vi "Self-Test.vi"(0 "VISA resource name":refnum<visa-resource-name>, 11 "error in (no error)":errorcluster {"code" format="%.0x"}) -> (4 "VISA resource name out":refnum<visa-resource-name>, 8 "Self-Test Result Code":i32, 10 "Self-Test Result Message":string, 15 "error out":errorcluster {"code" format="%.0x"})   [LabVIEW 2010, in "Agilent N6700 Series.lvlib"]
doc: "This VI runs the instrument's self test routine and returns the test results."
uses:
  Agilent N6700 Series.lvlib
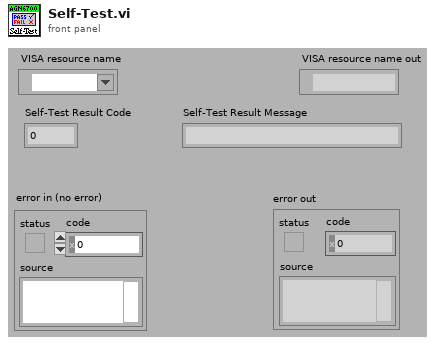
[diagram p1: front panel]
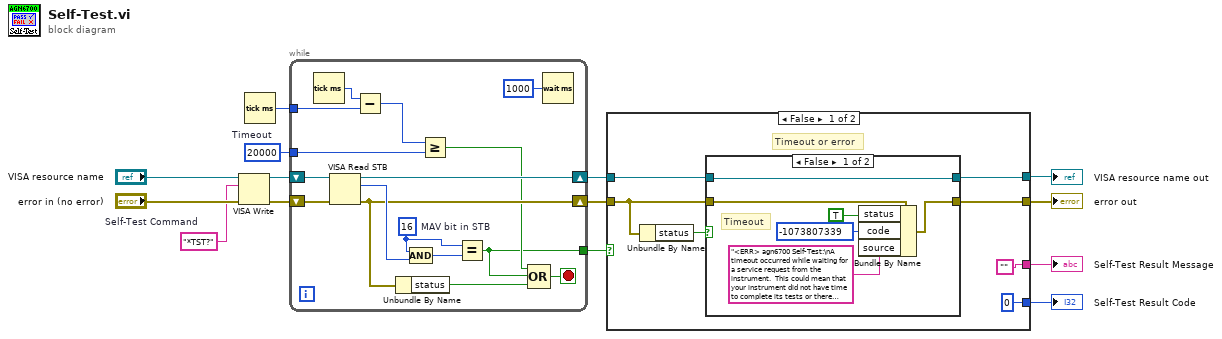
[diagram p0: block diagram]
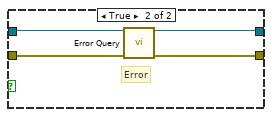
[diagram p2: hidden frame]
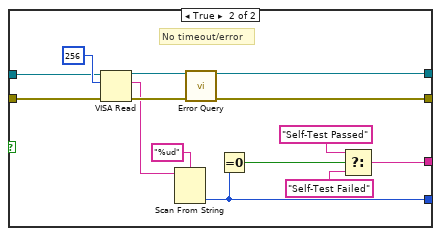
[diagram p3: hidden frame]
diagram:
  w2 = u32 20000  # Timeout
  w11 = "*TST?"  # Self-Test Command
  n1 = VISA Write(VISA resource name="VISA resource name", write buffer=w11, error in (no error)="error in (no error)") -> (VISA resource name out=w10:refnum<visa-resource-name>, error out=w9:errorcluster)  [unwired: 1 out]
  n2 = Tick Count (ms)() -> (millisecond timer value=w3:u32)
  n3 = while {
    shift-right: [w23] -> w7
    shift-left: w9 -> [w27]
    shift-right: [w25] -> w8
    shift-left: w10 -> [w26]
    tunnel: w3 -> [w19]
    tunnel: w2 -> [w17]
    tunnel: [w15] -> w1
    stop <- w21 stop-if-true
    w30 = u16 16  # MAV bit in STB
    n4 = Tick Count (ms)() -> (millisecond timer value=w20:u32)
    n5 = VISA Read STB(8:w27, 11:w26) -> (0:w23:errorcluster, 2:w28:u16, 3:w25:refnum<visa-resource-name>)
    n6 = Subtract(x=w20, y=w19) -> (x-y=w18:u32)
    n7 = Unbundle By Name(w23) -> ("status"=w22:bool)
    n8 = Compound Arithmetic op=AND(w30, w28) -> (w29:u16)
    n9 = Greater Or Equal?(x=w18, y=w17) -> (x >= y?=w16:bool)
    n10 = Equal?(x=w30, y=w29) -> (x = y?=w15:bool)
    n11 = Compound Arithmetic op=OR(w16, w15, w22) -> (w21:bool)
    n12 = Wait (ms)(milliseconds to wait=u32 1000) -> ()  [unwired: 1 out]
  }
  n13 = case shown="False" w1 {
    tunnel: ["" w48] -> w14
    tunnel: w8 -> [w36 w60]
    tunnel: w7 -> [w34 w59]
    tunnel: [0 w52] -> w6
    tunnel: [w35 w55] -> w5
    tunnel: [w33 w54] -> w4
    frame False {
      # "Timeout or error"
      n14 = Unbundle By Name(w34) -> ("status"=w37:bool)
      n15 = case shown="False" w37 {
        tunnel: w36 -> [w38 w47]
        tunnel: [w38 w44] -> w35
        tunnel: [w39 w45] -> w33
        tunnel: w34 -> [w40 w46]
        frame False {
          # "Timeout"
          n16 = Bundle By Name(cluster=w40, "status"=TRUE, "code"=-1073807339, "source"="<ERR> agn6700 Self-Test:\nA timeout occurred while waiting for a service request from the instrument.  This could mean that your instrument did not have time to complete its tests or there could be a problem communicating with the instrument.") -> (w39:errorcluster)
        }
        frame True {
          # "Error"
          n17 = call "Error Query.vi"("VISA resource name"=w47, "error in (no error)"=w46) -> ("VISA resource name out"=w44:refnum<visa-resource-name>, "error out"=w45:errorcluster)  [unwired: 10 in, 2 out]
        }
      }
    }
    frame True {
      # "No timeout/error"
      n18 = VISA Read(VISA resource name=w60, byte count=u32 256, error in (no error)=w59) -> (VISA resource name out=w56:refnum<visa-resource-name>, read buffer=w53:string, error out=w57:errorcluster)  [unwired: 1 out]
      n19 = Scan From String(format string="%ud", input string=w53) -> (output 1=w52:u32)  [unwired: 3 in, 3 out]
      n20 = call "Error Query.vi"("VISA resource name"=w56, "error in (no error)"=w57) -> ("VISA resource name out"=w55:refnum<visa-resource-name>, "error out"=w54:errorcluster)  [unwired: 10 in, 2 out]
      n21 = Equal To 0?(x=w52) -> (x = 0?=w51:bool)
      n22 = Select(t="Self-Test Passed" ("format string"), s=w51, f="Self-Test Failed" ("format string")) -> (s? t:f=w48:string)
    }
  }
  "Self-Test Result Message" <- w14
  "Self-Test Result Code" <- w6
  "VISA resource name out" <- w5
  "error out" <- w4
